vi "Clean Error Call Chain.vi"(8 "Error In":errorcluster) -> (0 "Error Out":errorcluster)   [LabVIEW 2018, in "LVH-LINX.lvlib"]
uses:
  LVH-LINX.lvlib
  <vilib>/regexp/Match Regular Expression.xnode
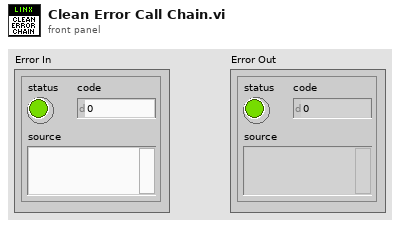
[diagram p1: front panel]
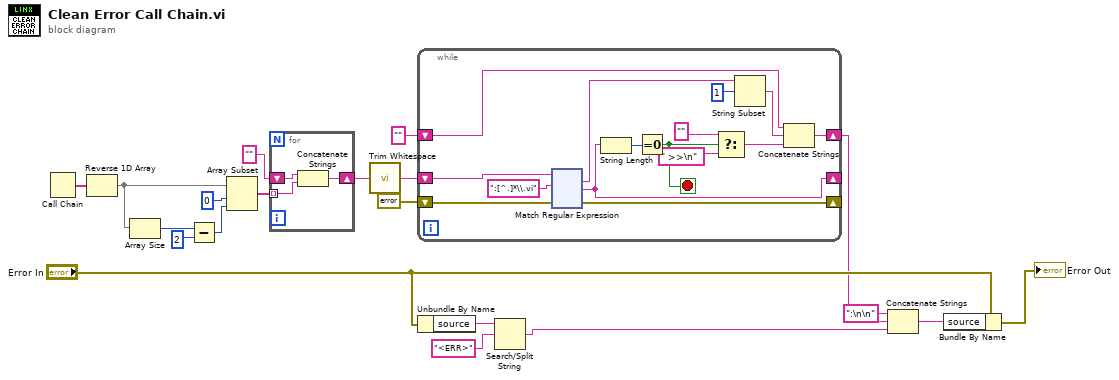
[diagram p0: block diagram]
diagram:
  n1 = Call Chain() -> (call chain=w13:string[])
  n2 = Reverse 1D Array(array=w13) -> (reversed array=w12:string[])
  n3 = Array Size(array=w12) -> (size(s)=w20:i32)
  n4 = Subtract(x=w20, y=2) -> (x-y=w18:i32)
  n5 = Array Subset(array=w12, index=0, length=w18) -> (w16:string[])
  n6 = for {
    tunnel: w16 -> [w22] mode=indexing
    shift-right: [w21] -> w9
    shift-left: "" -> [w23]
    n7 = Concatenate Strings(w23, w22) -> (w21:string)
  }
  n8 = call <vilib>:"Trim Whitespace.vi"("string"=w9) -> ("trimmed string"=w10:string)  [unwired: 1 in]
  n9 = while {
    shift-right: [w31] -> _
    shift-left: w10 -> [w38]
    shift-right: [w33] -> _
    shift-left: errorcluster {"status"=FALSE, "code"=0, "source"=""} ("error out") -> [w34]
    shift-right: [w27] -> w2
    shift-left: "" -> [w36]
    stop <- w29 stop-if-true
    n10 = xnode "Match Regular Expression"("input string"=w38, "regular expression"=":[^.]*\\.vi", "error in"=w34) -> ("whole match"=w26:string, "after match"=w31:string, "error out"=w33:errorcluster)  [unwired: 3 in, 2 out]
    n11 = String Length(string=w31) -> (length=w30:i32)
    n12 = Equal To 0?(x=w30) -> (x = 0?=w29:bool)
    n13 = Select(t="", s=w29, f=" >>\n" ("t")) -> (s? t:f=w28:string)
    n14 = String Subset(string=w26, offset (0)=1) -> (substring=w32:string)  [unwired: 1 in]
    n15 = Concatenate Strings(w36, w32, w28) -> (w27:string)
  }
  n16 = Unbundle By Name("Error In") -> ("source"=w6:string)
  n17 = Search/Split String(string=w6, search string/char (-)="<ERR>") -> (match + rest of string=w7:string)  [unwired: 1 in, 2 out]
  n18 = Concatenate Strings(":\n\n" ("string"), w2, w7) -> (w14:string)
  n19 = Bundle By Name(cluster="Error In", "source"=w14) -> (→"Error Out":errorcluster)
